vi "pointer.permute.advanced copy v2.vi"(8 "error in (no error)":errorcluster, 11 "TestCase in":refnum<class "TestCase.Pointer.lvclass">) -> (0 "error out":errorcluster, 2 "pass?":bool, 3 "TestCase out":refnum<class "TestCase.Pointer.lvclass">)   [LabVIEW 2016, in "TestCase.Pointer.lvclass"]
uses:
  TestCase.Pointer.lvclass
  TestCase.Pointer.lvclass/TestCase.Pointer.ctl
  Source/Classes/Pointer/Memory.Pointer.lvclass/Memory.Pointer.ctl
  Source/Classes/Pointer/Memory.Pointer.Write.Safe.0D.DBL.vi
  Source/Classes/Pointer/Memory.Pointer.Advanced Copy.Safe.vi
  Source/Classes/Pointer/Memory.Pointer.Read.Safe.0D.U8.vi
  Source/Classes/Pointer/Memory.Pointer.Read.Safe.0D.U16.vi
  Source/Classes/Pointer/Memory.Pointer.Read.Safe.0D.U32.vi
  Source/Classes/Pointer/Memory.Pointer.Read.Safe.0D.U64.vi
  Source/Classes/Pointer/Memory.Pointer.Write.Unsafe.0D.DBL.vi
  Source/Classes/Pointer/Memory.Pointer.Parameter Check.Null Pointer.vi
  Source/Classes/Pointer/Memory.Pointer.Parameter Check.Subset.vi
  Source/Classes/Pointer/Memory.Pointer.Advanced Copy.Unsafe.vi
  Source/Classes/Pointer/Memory.Pointer.Read.Unsafe.0D.U8.vi
  Source/Classes/Pointer/Memory.Pointer.Read.Unsafe.0D.U16.vi
  Source/Classes/Pointer/Memory.Pointer.Read.Unsafe.0D.U32.vi
  Source/Classes/Pointer/Memory.Pointer.Read.Unsafe.0D.U64.vi
  Source/Classes/Pointer/Memory.Pointer.Get Address.vi
  Source/Classes/Pointer/Memory.Pointer.Errors.vi
  Source/Classes/Pointer/Memory.Pointer.Errors.Null Pointer.vi
  Source/Classes/Pointer/Memory.Pointer.Errors.Out of Bounds.vi
  Source/Classes/Pointer/Memory.Pointer.Get Size.vi
  Source/Classes/Pointer/Memory.Pointer.Advanced Copy.Adjust Parameters.vi
  Source/Classes/Pointer/Memory.Pointer.Clear Subset.Unsafe.vi
  Source/Classes/Pointer/Memory.Pointer.Errors.Create Error.vi
  Source/Submodules/SEH/Source/VIs/Static Error Handling.Source Buffer.Write.String.vi
  Source/Classes/Pointer/Memory.Pointer.Errors.Write Pointer Size.vi
  Source/Submodules/SEH/Source/VIs/Static Error Handling.Source Buffer.Write.Numeric.Scalar.Base10.vi
  Source/Submodules/SEH/Source/VIs/Static Error Handling.Source Buffer.Write.Numeric.Scalar.Base10 (U64).vi
  Source/Submodules/SEH/Source/VIs/Static Error Handling.Error Cluster Constant.vi
  Source/Submodules/SEH/Source/VIs/Static Error Handling.Error Cluster Constant (256B).vi
  Source/Submodules/SEH/Source/VIs/Static Error Handling.Parameters.Status.Set.vi
  Source/Submodules/SEH/Source/VIs/Static Error Handling.Parameters.Code.Set.vi
  Source/Submodules/SEH/Source/VIs/Static Error Handling.Parameters.VI Source.Set.vi
  Source/Constants/Memory.Constants.vi
  Source/Constants/Memory.Constants.Library Name.vi
  Source/Classes/Pointer/Memory.Pointer.Errors.Get Info.vi
  Source/Classes/Internal/Memory.Pointer.Internal.lvclass
  C:/Users/Admin/Documents/LabVIEW-Memory/Source/Classes/Pointer/Memory.Pointer.lvclass
  Source/Classes/Pointer/Memory.Pointer.lvclass
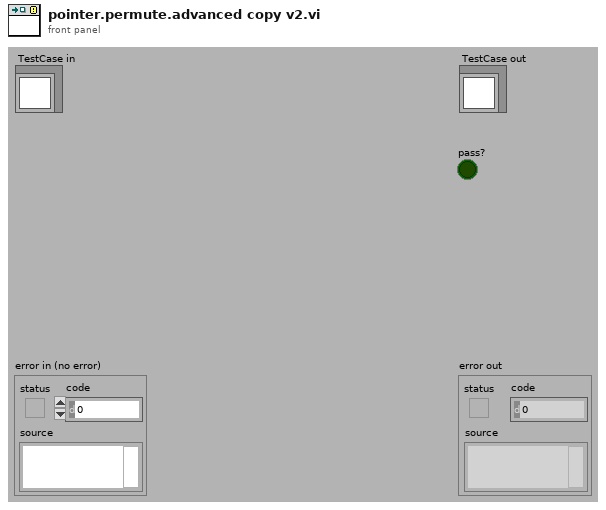
[diagram p1: front panel]
types:
  T1 = enum16{"big-endian, network order", "native, host order", "little-endian"}
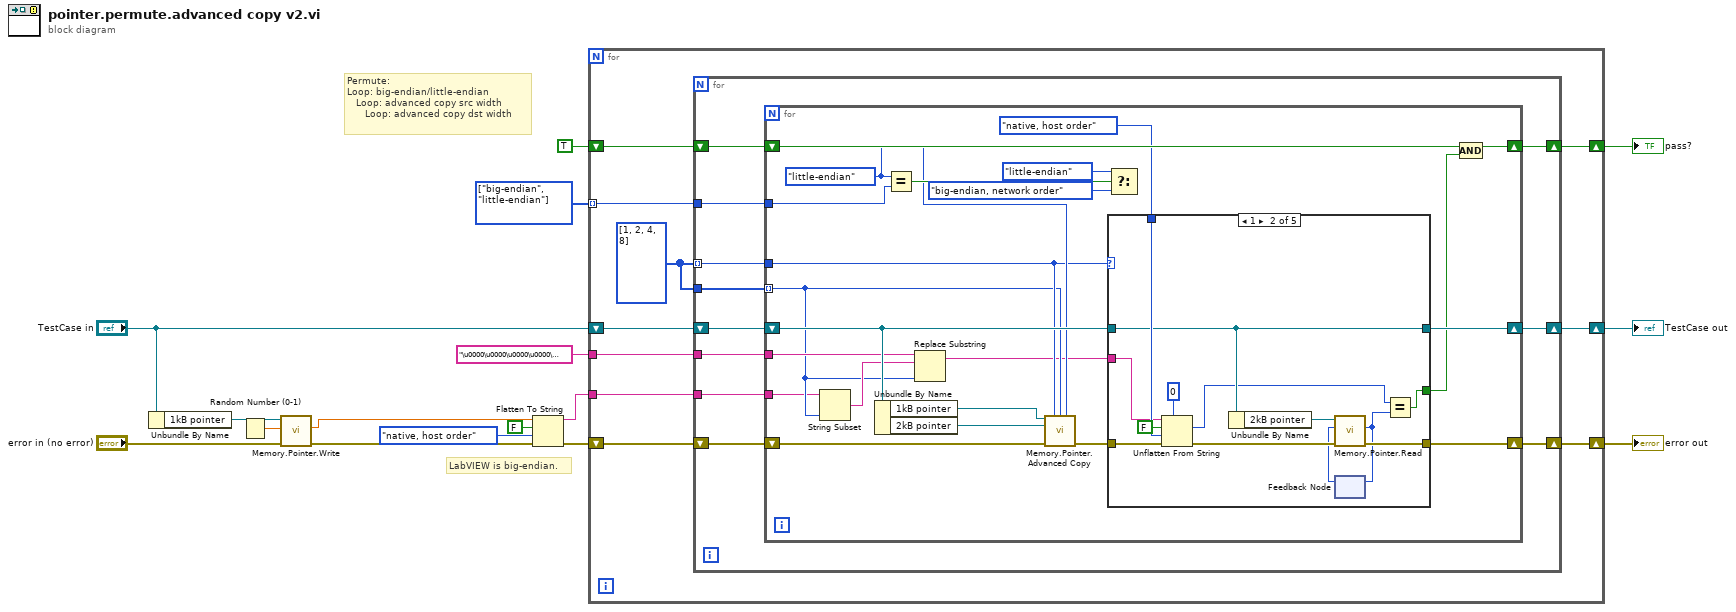
[diagram p0: block diagram]
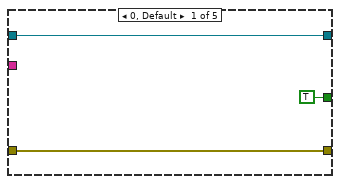
[diagram p2: hidden frame]
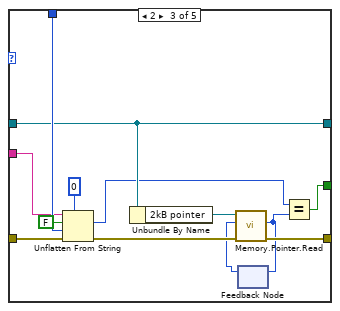
[diagram p3: hidden frame]
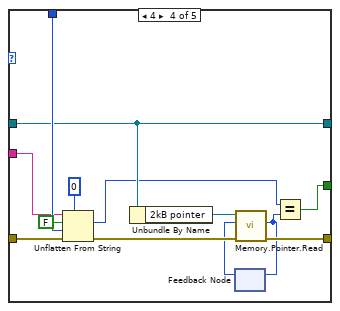
[diagram p4: hidden frame]
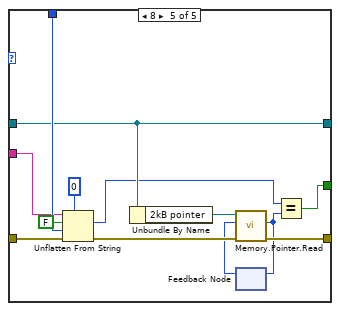
[diagram p5: hidden frame]
diagram:
  w16 = enum16{"big-endian", "little-endian"}[] [enum."big-endian", enum."little-endian"] items=["big-endian", "little-endian"] ("byte order (big-endian)")
  # "Permute:\nLoop: big-endian/little-endian\n   Loop: advanced copy src width\n      Loop: advanced copy dst width"
  # "LabVIEW is big-endian."
  n1 = Unbundle By Name("TestCase in") -> ("1kB pointer"=w15:refnum<class "Memory.Pointer.Internal.lvclass">)
  n2 = Random Number (0-1)() -> (number: 0 to 1=w14:dbl)
  n3 = call-poly "Memory.Pointer.Write.vi"("error in (no error)"="error in (no error)", "value"=w14, "pointer in"=w15) -> ("error out"=w12:errorcluster, "value"=w10:dbl)  [unwired: 5 in, 2 out]
  n4 = Flatten To String(anything=w10, prepend array or string size? (T)=FALSE, byte order (0:big-endian, network order)=T1."native, host order", error in (no error)=w12) -> (data string=w9:string, error out=w11:errorcluster)  [unwired: 1 out]
  n5 = for {
    shift-right: [w24] -> w4
    shift-left: w11 -> [w26]
    shift-right: [w23] -> w1
    shift-left: "TestCase in" -> [w25]
    tunnel: w16 -> [w21] mode=indexing
    tunnel: w9 -> [w20]
    shift-right: [w18] -> w7
    shift-left: TRUE -> [w19]
    tunnel: "\u0000\u0000\u0000\u0000\u0000\u0000\u0000\u0000" -> [w17]
    w22 = u64[] [1, 2, 4, 8] ("dst width")
    n6 = for {
      shift-right: [w34] -> w23
      shift-left: w25 -> [w36]
      shift-right: [w35] -> w24
      shift-left: w26 -> [w37]
      tunnel: w22 -> [w33] mode=indexing
      tunnel: w22 -> [w32]
      tunnel: w21 -> [w31]
      tunnel: w20 -> [w30]
      shift-right: [w28] -> w18
      shift-left: w19 -> [w29]
      tunnel: w17 -> [w27]
      n7 = for {
        shift-right: [w54] -> w34
        shift-left: w36 -> [w55]
        shift-right: [w53] -> w35
        shift-left: w37 -> [w45]
        tunnel: w33 -> [w41]
        tunnel: w32 -> [w40] mode=indexing
        tunnel: w31 -> [w49]
        tunnel: w30 -> [w39]
        shift-right: [w50] -> w28
        shift-left: w29 -> [w52]
        tunnel: w27 -> [w43]
        w44 = enum16{"big-endian", "little-endian"}."little-endian" ("byte order (big-endian)")
        n8 = String Subset(string=w39, length (rest)=w40) -> (substring=w42:string)  [unwired: 1 in]
        n9 = Unbundle By Name(w55) -> ("1kB pointer"=w48:refnum<class "Memory.Pointer.Internal.lvclass">, "2kB pointer"=w46:refnum<class "Memory.Pointer.Internal.lvclass">)
        n10 = Equal?(x=w44, y=w49) -> (x = y?=w59:bool)
        n11 = Replace Substring(2:w40, 4:w42, 5:w43) -> (1:w38:string)  [unwired: 1 in, 1 out]
        n12 = call-poly "Memory.Pointer.Advanced Copy.vi"("src pointer in"=w48, "dst width"=w41, "src width"=w40, "byte order (big-endian)"=w44, "dst pointer in"=w46, "error in (no error)"=w45) -> ("error out"=w56:errorcluster)  [unwired: 7 in, 2 out]
        n13 = case shown="1" w41 {
          tunnel: w56 -> [w61 w75 w88 w101 w114]
          tunnel: T1."native, host order" ("byte order (0:big-endian, network order)") -> [_ w74 w87 w100 w113]
          tunnel: w55 -> [w62 w72 w85 w98 w111]
          tunnel: [w62 w72 w85 w98 w111] -> w54
          tunnel: [w61 w69 w82 w95 w108] -> w53
          tunnel: [TRUE w65 w78 w91 w104] -> w51
          tunnel: w38 -> [_ w67 w80 w93 w106]
          frame 0, Default {
          }
          frame 1 {
            n14 = Unflatten From String(type=u8 0, binary string=w67, data includes array or string size? (T)=FALSE, byte order (0:big-endian, network order)=w74, error in (no error)=w75) -> (value=w66:u8, error out=w70:errorcluster)  [unwired: 1 out]
            n15 = Unbundle By Name(w72) -> ("2kB pointer"=w71:refnum<class "Memory.Pointer.Internal.lvclass">)
            n16 = feedback #1() -> (w64:u8)  [unwired: 1 in]
            n17 = call-poly "Memory.Pointer.Read.vi"("error in (no error)"=w70, "value in"=w64, "pointer in"=w71) -> ("error out"=w69:errorcluster, "value out"=w63:u8)  [unwired: 5 in, 2 out]
            n18 = feedback-in #1(w63) -> ()
            n19 = Equal?(x=w66, y=w63) -> (x = y?=w65:bool)
          }
          frame 2 {
            n20 = Unflatten From String(type=u16 0, binary string=w80, data includes array or string size? (T)=FALSE, byte order (0:big-endian, network order)=w87, error in (no error)=w88) -> (value=w79:u16, error out=w83:errorcluster)  [unwired: 1 out]
            n21 = Unbundle By Name(w85) -> ("2kB pointer"=w84:refnum<class "Memory.Pointer.Internal.lvclass">)
            n22 = feedback #2() -> (w76:u16)  [unwired: 1 in]
            n23 = call-poly "Memory.Pointer.Read.vi"("error in (no error)"=w83, "value in"=w76, "pointer in"=w84) -> ("error out"=w82:errorcluster, "value out"=w77:u16)  [unwired: 5 in, 2 out]
            n24 = feedback-in #2(w77) -> ()
            n25 = Equal?(x=w79, y=w77) -> (x = y?=w78:bool)
          }
          frame 4 {
            n26 = Unflatten From String(type=u32 0, binary string=w93, data includes array or string size? (T)=FALSE, byte order (0:big-endian, network order)=w100, error in (no error)=w101) -> (value=w92:u32, error out=w96:errorcluster)  [unwired: 1 out]
            n27 = Unbundle By Name(w98) -> ("2kB pointer"=w97:refnum<class "Memory.Pointer.Internal.lvclass">)
            n28 = feedback #3() -> (w89:u32)  [unwired: 1 in]
            n29 = call-poly "Memory.Pointer.Read.vi"("error in (no error)"=w96, "value in"=w89, "pointer in"=w97) -> ("error out"=w95:errorcluster, "value out"=w90:u32)  [unwired: 5 in, 2 out]
            n30 = feedback-in #3(w90) -> ()
            n31 = Equal?(x=w92, y=w90) -> (x = y?=w91:bool)
          }
          frame 8 {
            n32 = Unflatten From String(type=u64 0, binary string=w106, data includes array or string size? (T)=FALSE, byte order (0:big-endian, network order)=w113, error in (no error)=w114) -> (value=w105:u64, error out=w109:errorcluster)  [unwired: 1 out]
            n33 = Unbundle By Name(w111) -> ("2kB pointer"=w110:refnum<class "Memory.Pointer.Internal.lvclass">)
            n34 = feedback #4() -> (w102:u64)  [unwired: 1 in]
            n35 = call-poly "Memory.Pointer.Read.vi"("error in (no error)"=w109, "value in"=w102, "pointer in"=w110) -> ("error out"=w108:errorcluster, "value out"=w103:u64)  [unwired: 5 in, 2 out]
            n36 = feedback-in #4(w103) -> ()
            n37 = Equal?(x=w105, y=w103) -> (x = y?=w104:bool)
          }
        }
        n38 = Select(t=T1."little-endian" ("byte order (0:big-endian, network order)"), s=w59, f=T1."big-endian, network order" ("byte order (0:big-endian, network order)")) -> ()  [unwired: 1 out]
        n39 = Compound Arithmetic op=AND(w52, w51) -> (w50:bool)
      }
    }
  }
  "error out" <- w4
  "TestCase out" <- w1
  "pass?" <- w7
